vi "MakeErrorArray.vi"(11 "In":string) -> (2 "Out":string, 3 "ErrorArray":string[](array[string]))   [LabVIEW 2012]
panel:
  out "TimeStamp":string
  out "Reply":string
  out "Dir2":string
  out "Sent":string
  out "Dir1":string
  out "Success":string
  out "MethodName":string
  out "Error":string
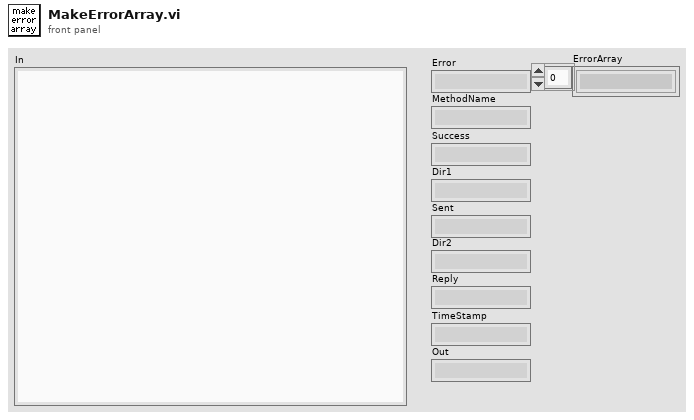
[diagram p1: front panel]
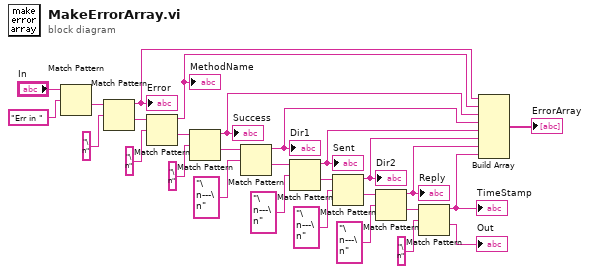
[diagram p0: block diagram]
diagram:
  n1 = Match Pattern(string="In", regular expression="Err in ") -> (after substring=w27:string)  [unwired: 1 in, 3 out]
  n2 = Match Pattern(string=w27, regular expression="\n") -> (before substring=w9:string, after substring=w23:string)  [unwired: 1 in, 2 out]
  "Error" <- w9
  n3 = Match Pattern(string=w23, regular expression="\n") -> (before substring=w8:string, after substring=w21:string)  [unwired: 1 in, 2 out]
  "MethodName" <- w8
  n4 = Match Pattern(string=w21, regular expression="\n") -> (before substring=w7:string, after substring=w19:string)  [unwired: 1 in, 2 out]
  "Success" <- w7
  n5 = Match Pattern(string=w19, regular expression="\n---\n") -> (before substring=w6:string, after substring=w17:string)  [unwired: 1 in, 2 out]
  "Dir1" <- w6
  n6 = Match Pattern(string=w17, regular expression="\n---\n") -> (before substring=w5:string, after substring=w13:string)  [unwired: 1 in, 2 out]
  "Sent" <- w5
  n7 = Match Pattern(string=w13, regular expression="\n---\n") -> (before substring=w4:string, after substring=w14:string)  [unwired: 1 in, 2 out]
  "Dir2" <- w4
  n8 = Match Pattern(string=w14, regular expression="\n---\n") -> (before substring=w3:string, after substring=w12:string)  [unwired: 1 in, 2 out]
  "Reply" <- w3
  n9 = Match Pattern(string=w12, regular expression="\n") -> (before substring=w2:string, after substring=→"Out":string)  [unwired: 1 in, 2 out]
  "TimeStamp" <- w2
  n10 = Build Array(w9, w8, w7, w6, w5, w4, w3, w2) -> (→"ErrorArray":string[])
